vi "svx_Timebase Update Data.vi"(6 "State in":T1={"X Scale"={"Name"="Time", "FString"="%#.2g", "Major Color"=16777238, "Minor Color"=16777216, "Grid Style"=1, "Maximum"=0.5, "Minimum"=0.0, "Autoscale"=TRUE, "Show Scale Label"={"Probe X"=FALSE, "Probe Y"=TRUE}, "Show Scale"={"Probe X"=TRUE, "Probe Y"=TRUE}, "Autoscale Once"=FALSE}, "Y Scale"={"Name"="Amplitude", "FString"="%#.2g", "Major Color"=16777238, "Minor Color"=16777216, "Scale Visible"=TRUE, " Label Visible"=TRUE, "Grid Style"=1, "Autoscale"=TRUE, "Maximum"={"Probe X"=1.0, "Probe Y"=1.0}, "Minimum"={"Probe X"=-1.0, "Probe Y"=-1.0}, "Autoscale Once"=FALSE}, "Plot"={"Point Style"=0, "Line Width"=0, "Line Style"=0, "Plot Color"=16860, "Point/fill"=16860}, "Tacho Point Color"=16711680, "Property Name"=[], "Container Bounds"={"Width"=640, "Height"=360}, "Background color"=16777226, "Legend Visible"=TRUE, "Scale Range Change"=refnum, "Strings[]"={"Custom pair name"=FALSE, "Row Strings []"=[], "Column Strings []"=[]}, "Cursor"={"Cursor Point Style"=13, "Cursor Style"=5, "Cursor Line Width"=1, "Cursor Line Style"=0, "Cursor Color"=16860, "Cursor Name Visible"=TRUE, "Cursor Visible"=TRUE, "Cursor Lock"=FALSE, "Cursor Index"=0}, "Index"=[], "Legend Width"=200, " Parents Tags"=[], "Children Tags"=[], "Open?"=[], "Label"="Timebase Plot", "Cursor X Pos"={"X"=0.0, "Y"=0.0}, "Cursor Y Pos"={"X"=0.0, "Y"=0.0}, "Graph Type"=enum."Probe X and Y", "Prev Graph Type"=enum."Probe X and Y", "Prev Legend Visible"=TRUE, "Cursor Release"=refnum, "Pair Strings Changed?"=FALSE, "Cursor ID"=refnum, "Legend Background"=16777226, "Legend Font"=16777222, "Probe Y Label"="Probe Y", "Probe X Label"="Probe X", "Probe X Label Visible"=TRUE, "Probe Y Label Visible"=TRUE, "Tree Item Width"=200, "# Custom RowStr"=0, "# Custom ColStr"=0, "Property Name"=refnum, "Data Related State"=refnum} caption="State", 7 "Data":T5, 9 "Probe Y":refnum<vi>, 10 "Probe X":refnum<vi>) -> (4 "State out":T1={"X Scale"={"Name"="Time", "FString"="%#.2g", "Major Color"=16777238, "Minor Color"=16777216, "Grid Style"=1, "Maximum"=0.5, "Minimum"=0.0, "Autoscale"=TRUE, "Show Scale Label"={"Probe X"=FALSE, "Probe Y"=TRUE}, "Show Scale"={"Probe X"=TRUE, "Probe Y"=TRUE}, "Autoscale Once"=FALSE}, "Y Scale"={"Name"="Amplitude", "FString"="%#.2g", "Major Color"=16777238, "Minor Color"=16777216, "Scale Visible"=TRUE, " Label Visible"=TRUE, "Grid Style"=1, "Autoscale"=TRUE, "Maximum"={"Probe X"=1.0, "Probe Y"=1.0}, "Minimum"={"Probe X"=-1.0, "Probe Y"=-1.0}, "Autoscale Once"=FALSE}, "Plot"={"Point Style"=0, "Line Width"=0, "Line Style"=0, "Plot Color"=16860, "Point/fill"=16860}, "Tacho Point Color"=16711680, "Property Name"=[], "Container Bounds"={"Width"=640, "Height"=360}, "Background color"=16777226, "Legend Visible"=TRUE, "Scale Range Change"=refnum, "Strings[]"={"Custom pair name"=FALSE, "Row Strings []"=[], "Column Strings []"=[]}, "Cursor"={"Cursor Point Style"=13, "Cursor Style"=5, "Cursor Line Width"=1, "Cursor Line Style"=0, "Cursor Color"=16860, "Cursor Name Visible"=TRUE, "Cursor Visible"=TRUE, "Cursor Lock"=FALSE, "Cursor Index"=0}, "Index"=[], "Legend Width"=200, " Parents Tags"=[], "Children Tags"=[], "Open?"=[], "Label"="Timebase Plot", "Cursor X Pos"={"X"=0.0, "Y"=0.0}, "Cursor Y Pos"={"X"=0.0, "Y"=0.0}, "Graph Type"=enum."Probe X and Y", "Prev Graph Type"=enum."Probe X and Y", "Prev Legend Visible"=TRUE, "Cursor Release"=refnum, "Pair Strings Changed?"=FALSE, "Cursor ID"=refnum, "Legend Background"=16777226, "Legend Font"=16777222, "Probe Y Label"="Probe Y", "Probe X Label"="Probe X", "Probe X Label Visible"=TRUE, "Probe Y Label Visible"=TRUE, "Tree Item Width"=200, "# Custom RowStr"=0, "# Custom ColStr"=0, "Property Name"=refnum, "Data Related State"=refnum} caption="State")   [LabVIEW 2017, in "SVX Timebase.xctl"]
uses:
  <vilib>/addons/_XControls/Timebase Plot/SVX Timebase.xctl
  <vilib>/addons/_XControls/Timebase Plot/subVIs/svx_Timebase Data.ctl
  <vilib>/addons/_XControls/Timebase Plot/subVIs/svx_Timebase State.ctl
  <vilib>/addons/_XControls/Timebase Plot/subVIs/svx_Timebase Bounds.ctl
  <vilib>/addons/_XControls/Timebase Plot/subVIs/svx_Timebase Graph Types.ctl
  <vilib>/addons/_XControls/Timebase Plot/subVIs/svx_Timebase Data Related State.ctl
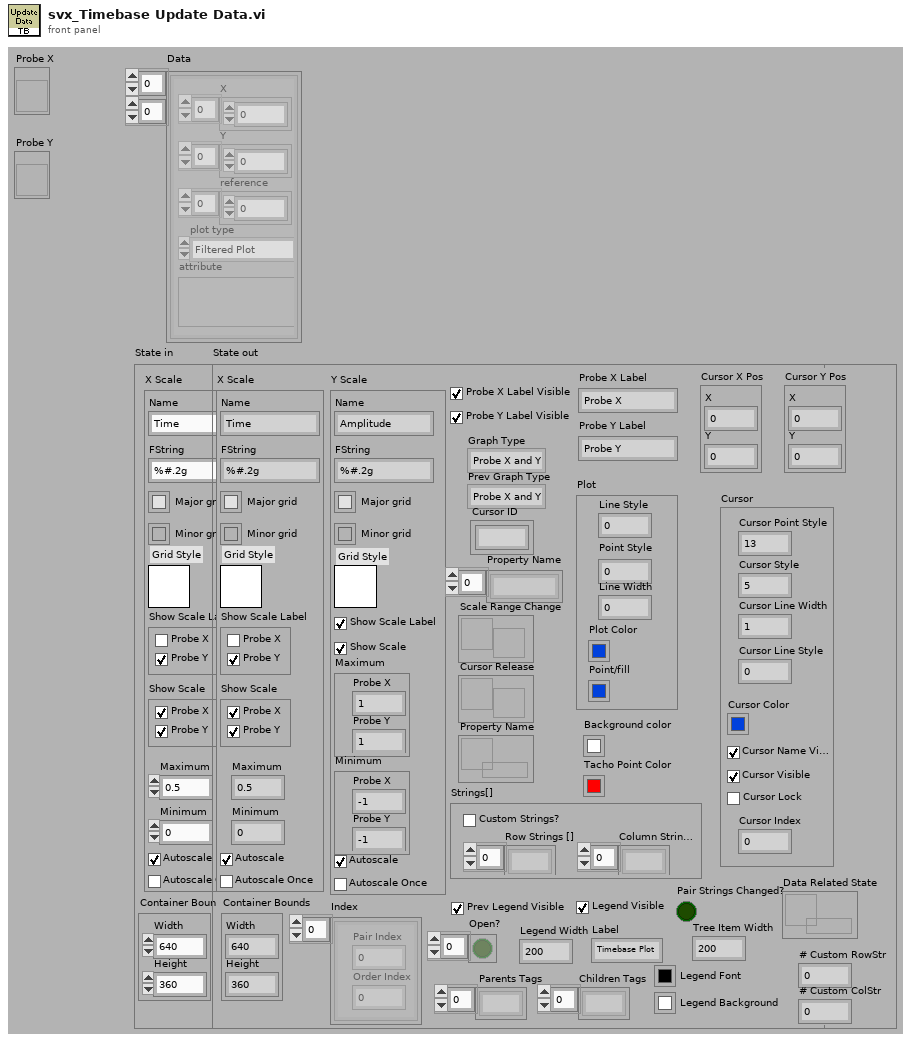
[diagram p1: front panel]
types:
  T1 = typedef "SVX Timebase.xctl/svx_Timebase State.ctl" = cluster{"X Scale":cluster{"Name":string, "FString":string, "Major Color":u32, "Minor Color":u32, "Grid Style":u16, "Maximum":dbl, "Minimum":dbl, "Autoscale":bool, "Show Scale Label":cluster{"Probe X":bool, "Probe Y":bool}, "Show Scale":cluster{"Probe X":bool, "Probe Y":bool}, "Autoscale Once":bool}, "Y Scale":cluster{"Name":string, "FString":string, "Major Color":u32, "Minor Color":u32, "Scale Visible":bool, " Label Visible":bool, "Grid Style":u16, "Autoscale":bool, "Maximum":cluster{"Probe X":dbl, "Probe Y":dbl}, "Minimum":cluster{"Probe X":dbl, "Probe Y":dbl}, "Autoscale Once":bool}, "Plot":cluster{"Point Style":u8, "Line Width":u8, "Line Style":u8, "Plot Color":u32, "Point/fill":u32}, "Tacho Point Color":u32, "Property Name":string[], "Container Bounds":T2, "Background color":u32, "Legend Visible":bool, "Scale Range Change":refnum<user-event>, "Strings[]":cluster{"Custom pair name":bool, "Row Strings []":string[], "Column Strings []":string[]}, "Cursor":cluster{"Cursor Point Style":u8, "Cursor Style":u8, "Cursor Line Width":u8, "Cursor Line Style":u8, "Cursor Color":u32, "Cursor Name Visible":bool, "Cursor Visible":bool, "Cursor Lock":bool, "Cursor Index":i32}, "Index":cluster{"Pair Index":u32, "Order Index":u32}[], "Legend Width":u32, " Parents Tags":string[], "Children Tags":string[], "Open?":bool[], "Label":string, "Cursor X Pos":cluster{"X":dbl, "Y":dbl}, "Cursor Y Pos":cluster{"X":dbl, "Y":dbl}, "Graph Type":T3, "Prev Graph Type":T3, "Prev Legend Visible":bool, "Cursor Release":refnum<user-event>, "Pair Strings Changed?":bool, "Cursor ID":refnum<k1>, "Legend Background":u32, "Legend Font":u32, "Probe Y Label":string, "Probe X Label":string, "Probe X Label Visible":bool, "Probe Y Label Visible":bool, "Tree Item Width":u32, "# Custom RowStr":u32, "# Custom ColStr":u32, "Property Name":refnum<queue>, "Data Related State":T4}
  T2 = typedef "SVX Timebase.xctl/svx_Timebase Bounds.ctl" = cluster{"Width":u32, "Height":u32}
  T3 = typedef "SVX Timebase.xctl/svx_Timebase Graph Types.ctl" = enum16{"Probe X", "Probe Y", "Probe X and Y"}
  T4 = typedef "SVX Timebase.xctl/svx_Timebase Data Related State.ctl" = refnum<queue>
  T5 = typedef "SVX Timebase.xctl/svx_Timebase Data.ctl" = cluster{"X":dbl[], "Y":dbl[], "reference":dbl[], "plot type":enum16{"Filtered Plot", "Unfiltered Plot"}, "attribute":variant}[][]
  T6 = cluster{"X":dbl[], "Y":dbl[], "reference":dbl[], "plot type":enum16{"Filtered Plot", "Unfiltered Plot"}, "attribute":variant}
  T7 = cluster{"orbit plot X":dbl[], "orbit plot Y":dbl[]}[]
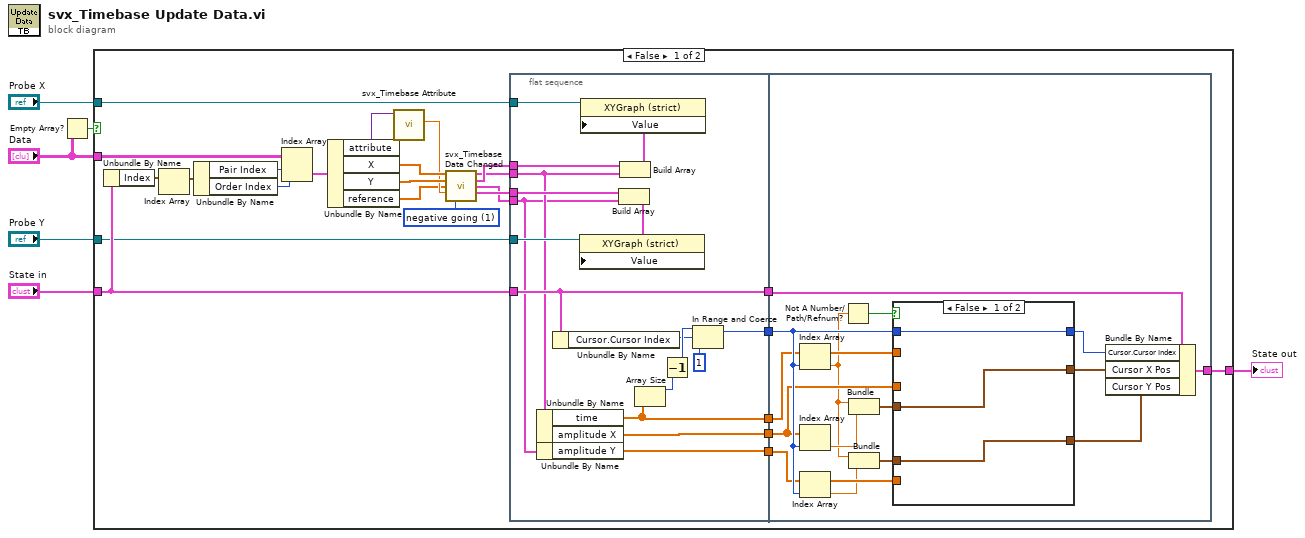
[diagram p0: block diagram]
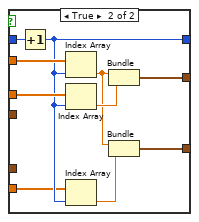
[diagram p2: hidden frame]
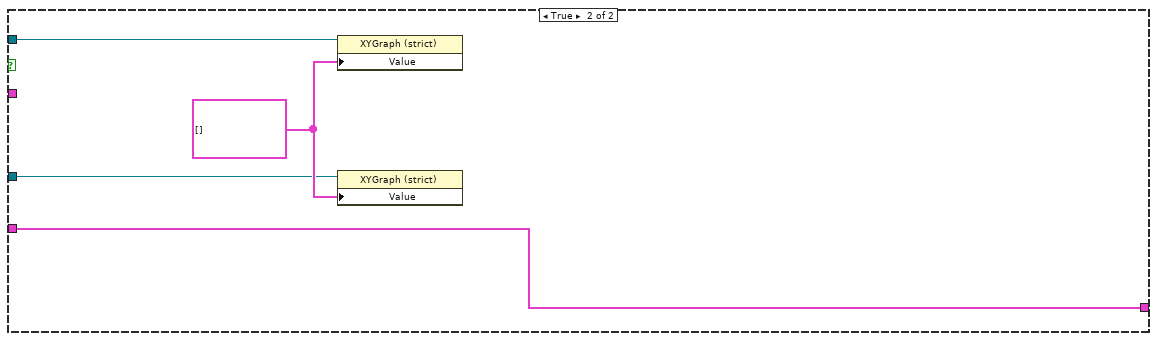
[diagram p3: hidden frame]
diagram:
  n1 = Empty Array?(array="Data") -> (empty?=w3:bool)
  n2 = case shown="False" w3 {
    tunnel: "State in" -> [w24 w80]
    tunnel: [w27 w80] -> w5
    tunnel: "Data" -> [w9 _]
    tunnel: "Probe X" -> [w18 w78]
    tunnel: "Probe Y" -> [w17 w77]
    frame False {
      w20 = u16 1 items=["positive going", "negative going"] ("trigger pulse direction")
      n3 = Unbundle By Name(w24) -> ("Index"=w25:cluster{"Pair Index":u32, "Order Index":u32}[])
      n4 = Index Array(array=w25) -> (element=w26:cluster{"Pair Index":u32, "Order Index":u32})  [unwired: 1 in]
      n5 = Unbundle By Name(w26) -> ("Pair Index"=w8:u32, "Order Index"=w7:u32)
      n6 = Index Array(array=w9, index (row)=w8, index (col)=w7) -> (element=w10:T6)
      n7 = Unbundle By Name(w10) -> ("attribute"=w28:variant, "X"=w30:dbl[], "Y"=w29:dbl[], "reference"=w22:dbl[])
      n8 = call <vilib>:"svx_Timebase Attribute.vi"("attribute"=w28) -> ("samples/rev"=w23:dbl)  [unwired: 8 in, 2 out]
      n9 = call <vilib>:"svx_Timebase Data Changed.vi"("X"=w30, "Y"=w29, "time reference"=w22, "actual samples/rev"=w23, "trigger pulse direction"=w20) -> ("probe X data"=w16:cluster{"time":dbl[], "amplitude X":dbl[]}, "tacho points X"=w19:cluster{dbl[], dbl[]}, "probe Y data"=w15:cluster{"time":dbl[], "amplitude Y":dbl[]}, "tacho points Y"=w21:cluster{dbl[], dbl[]})  [unwired: 7 in]
      n10 = flat-sequence {
        tunnel: w19 -> [w48]
        tunnel: w16 -> [w36]
        tunnel: [w42] -> w31
        tunnel: w24 -> [w42]
        tunnel: w21 -> [w47]
        tunnel: w15 -> [w35]
        tunnel: w18 -> [w46]
        tunnel: w17 -> [w45]
        tunnel: [w37] -> w14
        tunnel: [w34] -> w13
        tunnel: [w33] -> w12
        tunnel: [w32] -> w11
        tunnel: [w53] -> w27
        tunnel: w31 -> [w49]
        tunnel: w14 -> [w62]
        tunnel: w13 -> [w60]
        tunnel: w12 -> [w61]
        tunnel: w11 -> [w59]
        frame #0 {
          n11 = Unbundle By Name(w36) -> ("time"=w34:dbl[], "amplitude X"=w33:dbl[])
          n12 = Unbundle By Name(w35) -> ("amplitude Y"=w32:dbl[])
          n13 = Unbundle By Name(w42) -> ("Cursor.Cursor Index"=w38:i32)
          n14 = Build Array(w47, w35) -> (w43:cluster{"time":dbl[], "amplitude Y":dbl[]}[])
          n15 = property class="XYGraph (strict)"(reference=w45, "Value"=w43) -> ()  [unwired: 1 in, 2 out]
          n16 = Build Array(w48, w36) -> (w44:cluster{"time":dbl[], "amplitude X":dbl[]}[])
          n17 = property class="XYGraph (strict)"(reference=w46, "Value"=w44) -> ()  [unwired: 1 in, 2 out]
          n18 = Array Size(array=w34) -> (size(s)=w40:i32)
          n19 = Decrement(x=w40) -> (x-1=w39:i32)
          n20 = In Range and Coerce(upper limit=w39, x=w38, lower limit=1) -> (coerced(x)=w37:i32)  [unwired: 1 out]
        }
        frame #1 {
          n21 = Index Array(array=w60, index=w62) -> (element=w57:dbl)
          n22 = Index Array(array=w61, index=w62) -> (element=w58:dbl)
          n23 = Index Array(array=w59, index=w62) -> (element=w56:dbl)
          n24 = Not A Number/Path/Refnum?(number/path/refnum=w57) -> (NaN/Path/Refnum?=w63:bool)
          n25 = Bundle(w57, w58) -> (w55:cluster{dbl, dbl})  [unwired: 1 in]
          n26 = Bundle(w57, w56) -> (w54:cluster{dbl, dbl})  [unwired: 1 in]
          n27 = case shown="False" w63 {
            tunnel: w62 -> [w66 w72]
            tunnel: w60 -> [_ w76]
            tunnel: w61 -> [_ w75]
            tunnel: [w65 w73] -> w51
            tunnel: [w66 w71] -> w52
            tunnel: w59 -> [_ w70]
            tunnel: w55 -> [w65 _]
            tunnel: w54 -> [w64 _]
            tunnel: [w64 w67] -> w50
            frame False {
            }
            frame True {
              n28 = Increment(x=w72) -> (x+1=w71:i32)
              n29 = Index Array(array=w76, index=w71) -> (element=w69:dbl)
              n30 = Index Array(array=w75, index=w71) -> (element=w74:dbl)
              n31 = Index Array(array=w70, index=w71) -> (element=w68:dbl)
              n32 = Bundle(w69, w74) -> (w73:cluster{dbl, dbl})  [unwired: 1 in]
              n33 = Bundle(w69, w68) -> (w67:cluster{dbl, dbl})  [unwired: 1 in]
            }
          }
          n34 = Bundle By Name(cluster=w49, "Cursor.Cursor Index"=w52, "Cursor X Pos"=w51, "Cursor Y Pos"=w50) -> (w53:T1)
        }
      }
    }
    frame True {
      w79 = T7 [] ("Value (Signaling)")
      n35 = property on="Property Node" class="XYGraph (strict)"(reference=w78, "Value"=w79) -> ()  [unwired: 1 in, 2 out]
      n36 = property on="Property Node" class="XYGraph (strict)"(reference=w77, "Value"=w79) -> ()  [unwired: 1 in, 2 out]
    }
  }
  "State out" <- w5
